vi "Register New String Item.vi"(8 "error in (no error)":errorcluster, 9 "element data type":string, 10 "Tag Name":string, 11 "Current Value Table in":refnum<class "Current Value Table.lvclass">) -> (0 "error out":errorcluster, 3 "Current Value Table out":refnum<class "Current Value Table.lvclass">)   [LabVIEW 2024, in "Current Value Table.lvlib" / "Current Value Table.lvclass"]
uses:
  Current Value Table.lvclass
  CVT_String/CVT_String.lvclass
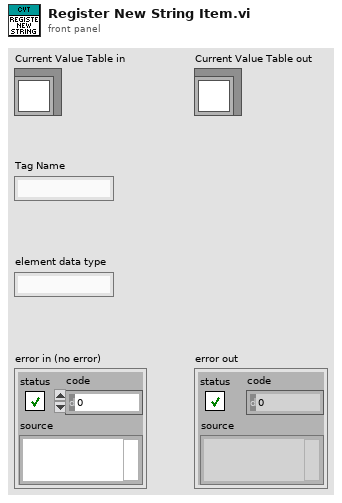
[diagram p1: front panel]
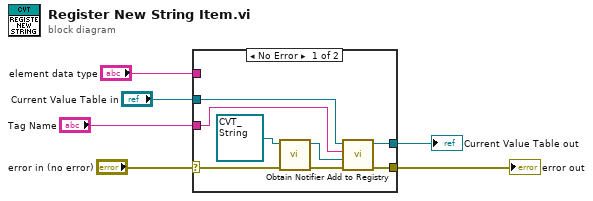
[diagram p0: block diagram]
diagram:
  n1 = case shown="No Error" "error in (no error)" {
    selector: "error in (no error)" -> [w8 w16]
    tunnel: [w10 w16] -> w5
    tunnel: [w9 w15] -> w3
    tunnel: "Current Value Table in" -> [w13 w15]
    tunnel: "element data type" -> [_ _]
    tunnel: "Tag Name" -> [w12 _]
    frame No Error {
      n2 = call-dynamic "Obtain Notifier.vi"("error in (no error)"=w8, "CVT_String in"=refnum<class "CVT_String.lvclass"> refnum) -> ("error out"=w7:errorcluster, "CVT_String out"=w11:refnum<class "CVT_String.lvclass">)  [unwired: 8 in]
      n3 = call-dynamic "Add to Registry.vi"("error in (no error)"=w7, "iCVT_Item in"=w11, "Tag Name"=w12, "Current Value Table in"=w13) -> ("error out"=w10:errorcluster, "Current Value Table out"=w9:refnum<class "Current Value Table.lvclass">)  [unwired: 5 in, 1 out]
    }
    frame Error {
    }
  }
  "error out" <- w5
  "Current Value Table out" <- w3
